vi "PostResult.vi"(8 "error in (no error)":errorcluster, 11 "reference in":refnum<class "Test_Template.lvclass">) -> (0 "error out":errorcluster, 1 "Pass":bool, 3 "reference in":refnum<class "Test_Template.lvclass">)   [LabVIEW 2017]
uses:
  Test_Template.lvclass
  Components/MES_Base.lvlibp/MES_Base.lvclass
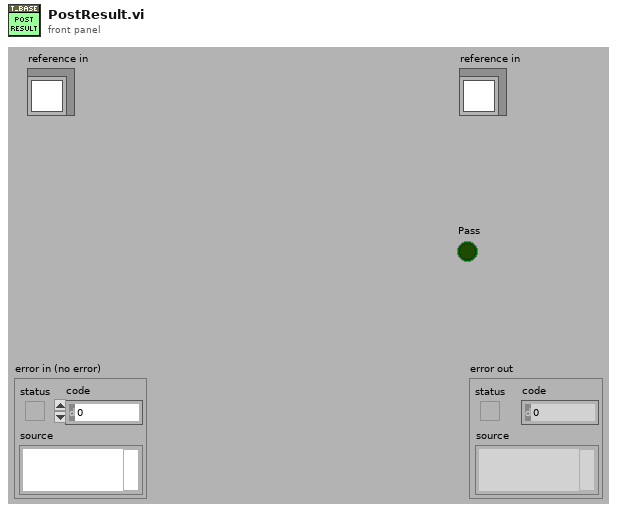
[diagram p1: front panel]
types:
  T1 = typedef "Test_Template.lvlib/Test_Template.lvclass/ObjectAttributes.ctl" = cluster{"Config":T2}
  T2 = typedef "Test_Template.lvlib/Test_Template.lvclass/Config.ctl" = cluster{"default":string}
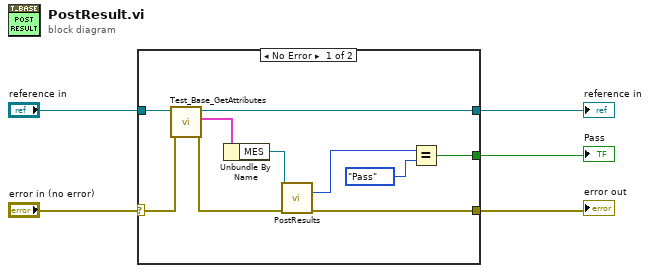
[diagram p0: block diagram]
diagram:
  n1 = case shown="No Error" "error in (no error)" {
    selector: "error in (no error)" -> [w15 w17]
    tunnel: [w11 w17] -> w4
    tunnel: [w9 w16] -> w2
    tunnel: "reference in" -> [w13 w16]
    tunnel: [w6 _] -> w1
    frame No Error {
      n2 = call "Test_Base_GetAttributes.vi"("error in (no error)"=w15, "reference in"=w13) -> ("error out"=w10:errorcluster, "Data"=w14:T1, "reference out"=w9:refnum<class "Test_Template.lvclass">)  [unwired: 6 in, 1 out]
      n3 = Unbundle By Name(w14) -> ("MES"=w12:refnum<class "MES_Base.lvclass">)
      n4 = call-dynamic "PostResults.vi"("reference in"=w12, "error in (no error)"=w10) -> ("Result"=w8:enum16{"Pending", "Pass", "Fail"}, "error out"=w11:errorcluster)  [unwired: 11 in, 1 out]
      n5 = Equal?(x=w8, y=enum16{"Pending", "Pass", "Fail"}."Pass") -> (x = y?=w6:bool)
    }
    frame Error {
    }
  }
  "error out" <- w4
  "reference in" <- w2
  "Pass" <- w1
